vi "rp_explore.vi"(6 "Variant in":variant, 7 "Shift Pressed?":bool, 8 "error in (no error)":errorcluster, 10 "QD Combo Box Ref":refnum<vi>, 11 "QD Launch VI Ref":refnum<vi>) -> (0 "error out":errorcluster, 4 "Variant out":variant)   [LabVIEW 2019]
doc: "Open in file explorer.\n\nCreated by: Ryan Pacini\n\nDefault Shortcut - [0]"
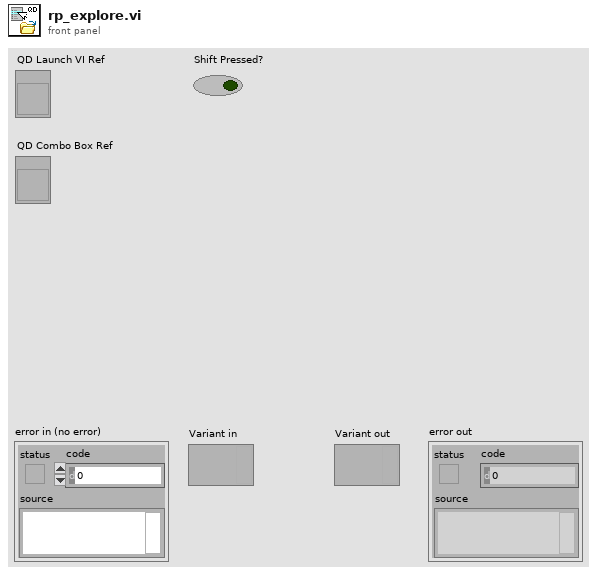
[diagram p1: front panel]
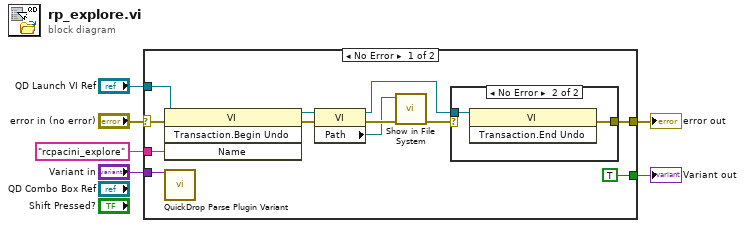
[diagram p0: block diagram]
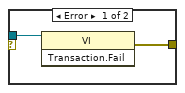
[diagram p2: hidden frame]
diagram:
  n1 = case shown="No Error" "error in (no error)" {
    selector: "error in (no error)" -> [w18 w23]
    tunnel: [w17 w23] -> w2
    tunnel: "QD Launch VI Ref" -> [w14 _]
    tunnel: "rcpacini_explore" ("Undo Name") -> [w16 _]
    tunnel: [TRUE _] -> w3
    tunnel: "Variant in" -> [w7 _]
    frame No Error {
      n2 = invoke class="VI" method="Transaction.Begin Undo"(reference=w14, error in=w18, "Name"=w16) -> (reference out=w12:refnum<vi>, error out=w13:errorcluster)  [unwired: 1 in, 2 out]
      n3 = call <vilib>:"QuickDrop Parse Plugin Variant.vi"("QDKS Variant in"=w7) -> ()  [unwired: 12 in, 3 out]
      n4 = property class="VI"(reference=w12, error in=w13) -> (reference out=w8:refnum<vi>, error out=w11:errorcluster, "Path"=w10:path)
      n5 = call <vilib>:"Show in File System.vi"("error in (no error)"=w11, "file or directory path"=w10) -> ("error out"=w9:errorcluster)  [unwired: 9 in]
      n6 = case shown="No Error" w9 {
        tunnel: w8 -> [w19 w21]
        tunnel: [w20 w22] -> w17
        frame Error {
          n7 = invoke class="VI" method="Transaction.Fail"(reference=w19) -> (error out=w20:errorcluster)  [unwired: 2 in, 2 out]
        }
        frame No Error {
          n8 = invoke class="VI" method="Transaction.End Undo"(reference=w21) -> (error out=w22:errorcluster)  [unwired: 2 in, 2 out]
        }
      }
    }
    frame Error {
    }
  }
  "error out" <- w2
  "Variant out" <- w3
